vi "Get or Create Sub Object.vi"(8 "error in":errorcluster, 10 "Sub Index":u8 format="%.0x", 11 "Obj Entry in":refnum<class "Object Entry.lvclass">) -> (0 "error out":errorcluster, 1 "Sub Object":refnum<class "Sub Object.lvclass">, 3 "Obj Entry out":refnum<class "Object Entry.lvclass">)   [LabVIEW 2020, in "CANopen.lvlib" / "Object Entry.lvclass"]
uses:
  Object Entry.lvclass
  Object Entry.lvclass/Object Entry.ctl
  Sub Objects Dictionary/Sub Objects Dictionary.lvclass
  Sub Object/Sub Object.lvclass
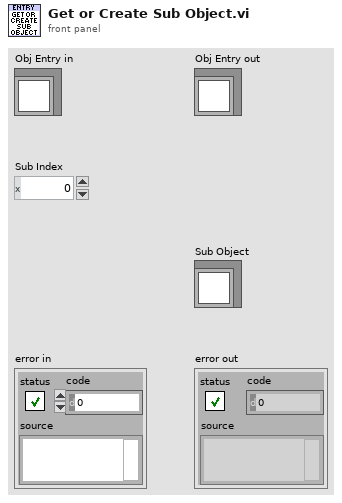
[diagram p1: front panel]
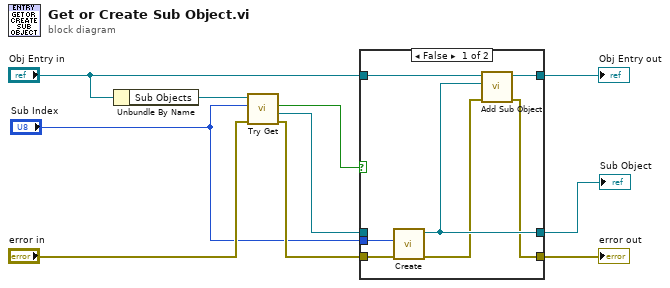
[diagram p0: block diagram]
diagram:
  n1 = Unbundle By Name("Obj Entry in") -> ("Sub Objects"=w10:refnum<class "Sub Objects Dictionary.lvclass">)
  n2 = call "Try Get.vi"("error in"="error in", "Sub Index"="Sub Index", "Sub Objects Dictionary in"=w10) -> ("error out"=w8:errorcluster, "Sub Obj"=w5:refnum<class "Sub Object.lvclass">, "Success"=w6:bool)  [unwired: 5 in, 1 out]
  n3 = case shown="False" w6 {
    tunnel: w8 -> [w17 w20]
    tunnel: [w12 w20] -> w7
    tunnel: w5 -> [_ w19]
    tunnel: "Sub Index" -> [w16 _]
    tunnel: [w14 w19] -> w3
    tunnel: "Obj Entry in" -> [w15 w18]
    tunnel: [w11 w18] -> w1
    frame False {
      n4 = call "Create.vi"("error in"=w17, "Sub Index"=w16) -> ("error out"=w13:errorcluster, "Sub Obj out"=w14:refnum<class "Sub Object.lvclass">)  [unwired: 8 in]
      n5 = call "Add Sub Object.vi"("error in"=w13, "Sub Object"=w14, "Obj Entry in"=w15) -> ("error out"=w12:errorcluster, "Obj Entry out"=w11:refnum<class "Object Entry.lvclass">)  [unwired: 7 in]
    }
    frame True {
    }
  }
  "error out" <- w7
  "Obj Entry out" <- w1
  "Sub Object" <- w3
